vi "Close.vi"(8 "error in (no error)":errorcluster, 11 "EventFile in":refnum<class "EventFile.lvclass">) -> (0 "error out":errorcluster)   [LabVIEW 2016, in "Event Logging.lvlib" / "EventFile.lvclass"]
uses:
  EventFile.lvclass
  EventFile.lvclass/EventFile.ctl
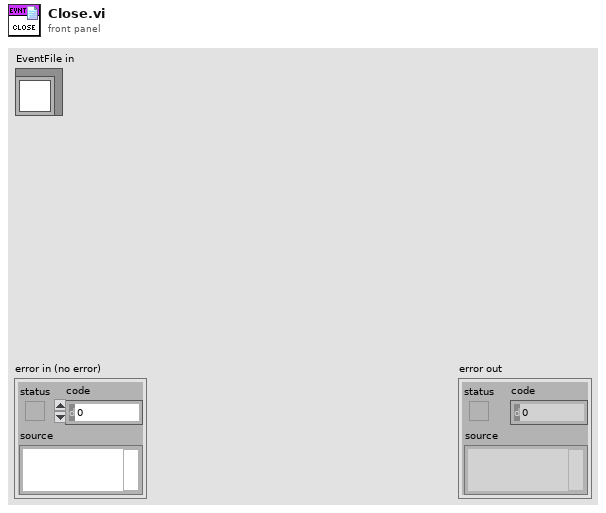
[diagram p1: front panel]
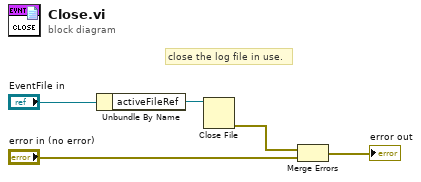
[diagram p0: block diagram]
diagram:
  # "close the log file in use."
  n1 = Unbundle By Name("EventFile in") -> ("activeFileRef"=w4:refnum<file>)
  n2 = Close File(refnum=w4) -> (error out=w3:errorcluster)  [unwired: 1 in, 1 out]
  n3 = Merge Errors(w3, "error in (no error)") -> (→"error out":errorcluster)
